vi "Begin.vi"(8 "error in":errorcluster) -> (0 "error out":errorcluster)   [LabVIEW 2019]
doc: "Called before other user functions, this VI is expected to open initial I/O refnums, load in file data, and do all program initialization. Notice that the <B>error out</B> terminal is simply used for data flow. Wiring it to other structures or subVIs ensures that this VI runs first."
uses:
  <vilib>/Rock Robotics/WPI/DriverStation/WPI_DriverStationRobotMode2.ctl
  <vilib>/Rock Robotics/WPI/Joystick/WPI_JoystickDeviceEnum.ctl
  <vilib>/Rock Robotics/SystemInterfaces/DIO/FPGA_DIOChannel.ctl
  <vilib>/Rock Robotics/WPI/Encoder/WPI_EncoderType.ctl
  <vilib>/Rock Robotics/WPI/ThirdParty/REV Robotics/SPARK MAX/Typedef/Spark MAX Motor Type.ctl
  <vilib>/Rock Robotics/WPI/ThirdParty/REV Robotics/SPARK MAX/Typedef/Spark MAX Idle Mode.ctl
  <vilib>/Rock Robotics/WPI/SafetyOutput/WPI_SafetyOutputConfigMenu.ctl
  <vilib>/Rock Robotics/WPI/ThirdParty/Phoenix-LabVIEW/Motor Controller/Controls/CTRE_Phoenix_MotorControl_ControlMode.ctl
  <vilib>/Rock Robotics/WPI/Solenoid/WPI_SolenoidChannel.ctl
  Robot Global Data.vi
  <vilib>/Rock Robotics/Network Tables/NT Write String Array.vi
  <vilib>/Rock Robotics/WPI/Counter/WPI_CounterDigitalInputToDigitalSource.vi
  <vilib>/Rock Robotics/WPI/RobotDrive/WPI_RobotDriveOpen4MotorWithExistingMotors.vi
  <vilib>/Rock Robotics/WPI/Solenoid/WPI_SolenoidOpenDouble.vi
  <vilib>/Rock Robotics/WPI/Switch/WPI_SwitchOpenLimit.vi
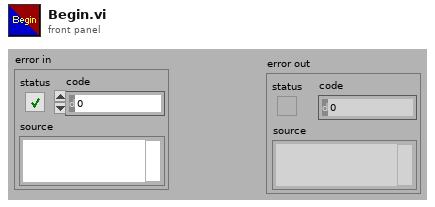
[diagram p1: front panel]
types:
  T1 = typedef "FPGA_DIOChannel.ctl" = enum8{"DIO 0", "DIO 1", "DIO 2", "DIO 3", "DIO 4", "DIO 5", "DIO 6", "DIO 7", "DIO 8", "DIO 9", "DIO MXP 0", "DIO MXP 1", "DIO MXP 2", "DIO MXP 3", "DIO MXP 4", "DIO MXP 5", "DIO MXP 6", "DIO MXP 7", "DIO MXP 8", "DIO MXP 9", "DIO MXP 10", "DIO MXP 11", "DIO MXP 12", "DIO MXP 13", "DIO MXP 14", "DIO MXP 15", "SPI Port CS1", "SPI Port CS2", "SPI Port CS3", "SPI Port MISO", "SPI Port MOSI", "Invalid"}
  T2 = typedef "CTRE_Phoenix_MotorControl_ControlMode.ctl" = u16
  T3 = typedef "WPI_SolenoidChannel.ctl" = enum8{"Solenoid 0", "Solenoid 1", "Solenoid 2", "Solenoid 3", "Solenoid 4", "Solenoid 5", "Solenoid 6", "Solenoid 7", "Invalid"}
  T4 = typedef "WPI_SafetyOutputConfigMenu.ctl" = enum16{"Enable", "Disable"}
  T5 = typedef "Spark MAX Idle Mode.ctl" = enum16{"Coast", "Brake"}
  T6 = typedef "Spark MAX Motor Type.ctl" = enum16{"Brushed", "Brushless"}
  T7 = typedef "WPI_EncoderType.ctl" = enum16{"1x", "2x", "4x"}
  T8 = typedef "WPI_JoystickDeviceEnum.ctl" = enum16{"USB 0", "USB 1", "USB 2", "USB 3", "USB 4", "USB 5"}
  T9 = typedef "WPI_DriverStationRobotMode2.ctl" = enum16{"Autonomous Disabled", "Autonomous Enabled", "Teleop Disabled", "Teleop Enabled", "Disconnected", "Finish", "Test Disabled", "Test Enabled", "Emergency Stopped"}
  T10 = typedef "WPI_SwitchDevRef.ctl" = cluster{"DevStatus":errorcluster, "DIO Channel":T1, "CntIndex":T11, "Normally Closed":bool}
  T11 = typedef "FPGA_CounterCtrSystemIndex.ctl" = enum8{"Ctr 0", "Ctr 1", "Ctr 2", "Ctr 3", "Ctr 4", "Ctr 5", "Ctr 6", "Ctr 7", "Invalid"}
  T12 = typedef "WPI_MotorControlDeviceRef.ctl" = cluster{"DeviceStatus":errorcluster, "Type":T13, "PWM":cluster{"PWM Channel":T14, "DeadBand":T15}, "CAN":cluster{"Device Number":u8, "SetOutput VI Ref":variant, "GetOutput VI Ref":variant, "Enable VI Ref":variant, "Disable VI Ref":variant, "Data":variant}, "Invert":bool, "DIO PWM":cluster{"PWM \"Enable\" Channel":T14, "DIOChannel":T1, "PWM Rate":dbl}}
  T13 = typedef "WPI_MotorControlType.ctl" = enum16{"PWM", "CAN", "DIO PWM"}
  T14 = typedef "FPGA_DIOPWMChannel.ctl" = enum8{"PWM 0", "PWM 1", "PWM 2", "PWM 3", "PWM 4", "PWM 5", "PWM 6", "PWM 7", "PWM 8", "PWM 9", "PWM MXP 0", "PWM MXP 1", "PWM MXP 2", "PWM MXP 3", "PWM MXP 4", "PWM MXP 5", "PWM MXP 6", "PWM MXP 7", "PWM MXP 8", "PWM MXP 9", "Invalid"}
  T15 = typedef "WPI_PWMDeadband.ctl" = cluster{"Name":string, "maxPositivePwm":i32, "minPositivePwm":i32, "centerPwm":i32, "maxNegativePwm":i32, "minNegativePwm":i32, "angularRange":u16}
  T16 = typedef "WPI_JoystickDevRef.ctl" = cluster{"Device":T8}
  T17 = typedef "WPI_RobotDriveDevRef.ctl" = cluster{"DevStatus":errorcluster, "Motors[]":T12[], "Square Inputs":bool, "Max Output":dbl}
  T18 = typedef "WPI_SolenoidDevRef.ctl" = cluster{"DevStatus":errorcluster, "Pneumatics Control Module":u8, "Forward Solenoid Channel":T3, "Reverse Solenoid Channel":T3}
  T19 = typedef "WPI_DigitalInputDevRef.ctl" = cluster{"DevStatus":errorcluster, "DIO Channel":T1}
  T20 = typedef "FPGA_CounterEncoderSourceConvertionLVSourceType.ctl" = cluster{"DevStatus":errorcluster, "AnalogTriggerMode?":bool, "DigitalMode":cluster{"DIO Channel":T21}, "AnalogTriggerMode":cluster{"AnalogTriggerIndex":T22, "OutputType":T23}}
  T21 = typedef "FPGA_DIODigitalSourceChannel.ctl" = enum8{"DIO 0", "DIO 1", "DIO 2", "DIO 3", "DIO 4", "DIO 5", "DIO 6", "DIO 7", "DIO 8", "DIO 9", "DIO MXP 0", "DIO MXP 1", "DIO MXP 2", "DIO MXP 3", "DIO MXP 4", "DIO MXP 5", "DIO MXP 6", "DIO MXP 7", "DIO MXP 8", "DIO MXP 9", "DIO MXP 10", "DIO MXP 11", "DIO MXP 12", "DIO MXP 13", "DIO MXP 14", "DIO MXP 15", "SPI Port CS1", "SPI Port CS2", "SPI Port CS3", "SPI Port MISO", "SPI Port MOSI", "Disabled"}
  T22 = typedef "FPGA_AnalogTriggerIndex.ctl" = enum8{"Trig 0", "Trig 1", "Trig 2", "Trig 3", "Trig 4", "Trig 5", "Trig 6", "Trig 7", "Invalid"}
  T23 = typedef "FPGA_AnalogTriggerOutType.ctl" = enum16{"InWindow", "TriggerState", "Rising", "Falling"}
  T24 = typedef "WPI_EncoderDevRef.ctl" = cluster{"DevStatus":errorcluster, "EncoderIndex":T25, "CounterIndex":T11, "DistancePerCount":dbl, "Decoding Type":T7}
  T25 = typedef "FPGA_EncoderIdx.ctl" = enum8{"Enc 0", "Enc 1", "Enc 2", "Enc 3", "Enc 4", "Enc 5", "Enc 6", "Enc 7", "Invalid"}
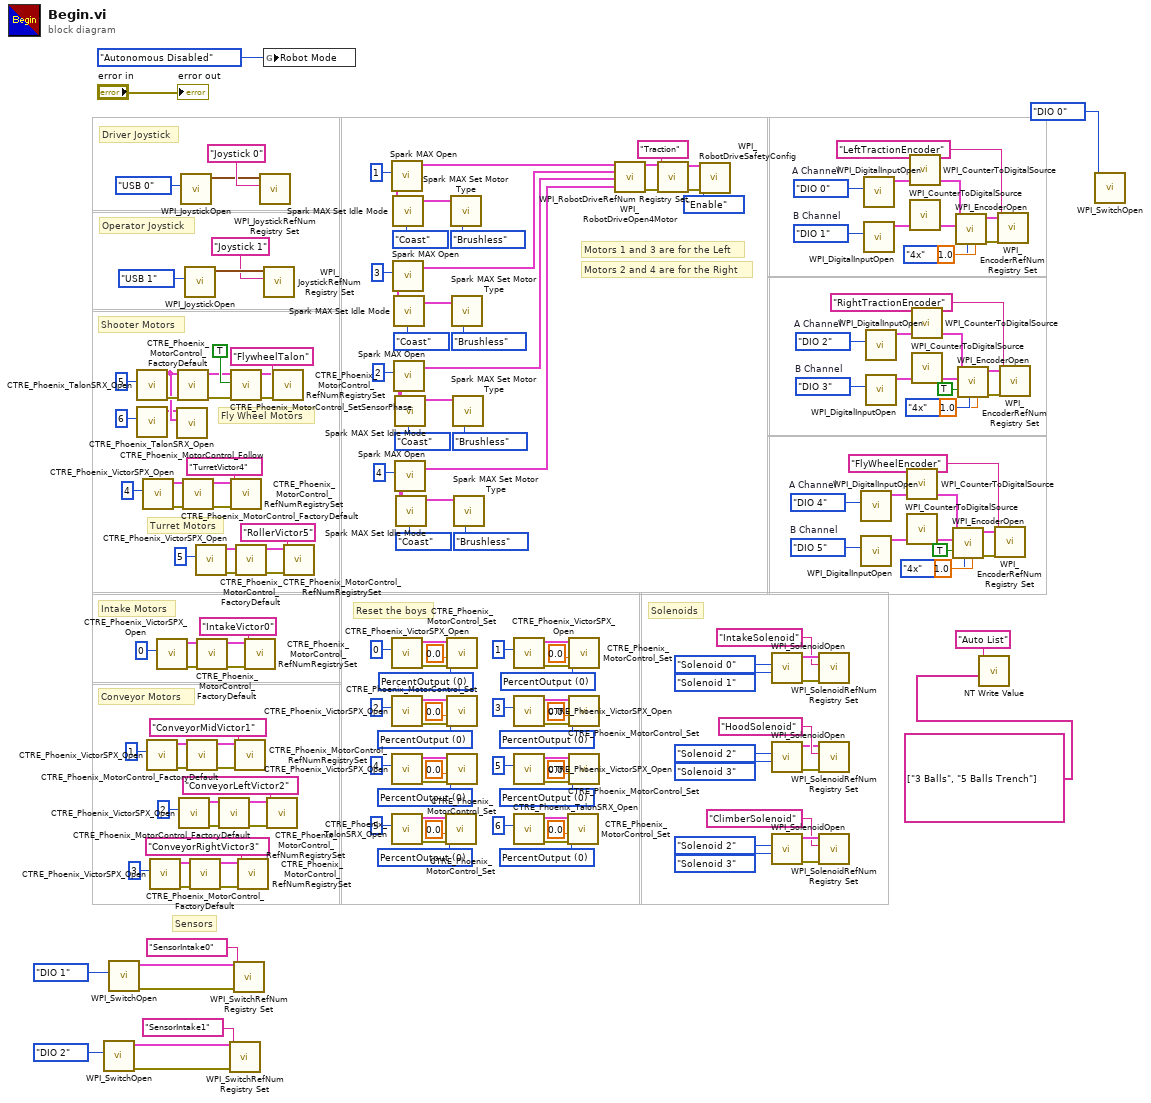
[diagram p0: block diagram]
diagram:
  w11 = T2 0 items=["PercentOutput"=0, "Position"=1, "Velocity"=2, "Current"=3, "Follower"=5, "MotionProfile"=6, "MotionMagic"=7, "MotionMagicArc"=8, "MotionProfileArc"=10, "Disabled"=15] ("Control Mode")
  w35 = T2 0 items=["PercentOutput"=0, "Position"=1, "Velocity"=2, "Current"=3, "Follower"=5, "MotionProfile"=6, "MotionMagic"=7, "MotionMagicArc"=8, "MotionProfileArc"=10, "Disabled"=15] ("Control Mode")
  w41 = T2 0 items=["PercentOutput"=0, "Position"=1, "Velocity"=2, "Current"=3, "Follower"=5, "MotionProfile"=6, "MotionMagic"=7, "MotionMagicArc"=8, "MotionProfileArc"=10, "Disabled"=15] ("Control Mode")
  w40 = T2 0 items=["PercentOutput"=0, "Position"=1, "Velocity"=2, "Current"=3, "Follower"=5, "MotionProfile"=6, "MotionMagic"=7, "MotionMagicArc"=8, "MotionProfileArc"=10, "Disabled"=15] ("Control Mode")
  w50 = T2 0 items=["PercentOutput"=0, "Position"=1, "Velocity"=2, "Current"=3, "Follower"=5, "MotionProfile"=6, "MotionMagic"=7, "MotionMagicArc"=8, "MotionProfileArc"=10, "Disabled"=15] ("Control Mode")
  w51 = T2 0 items=["PercentOutput"=0, "Position"=1, "Velocity"=2, "Current"=3, "Follower"=5, "MotionProfile"=6, "MotionMagic"=7, "MotionMagicArc"=8, "MotionProfileArc"=10, "Disabled"=15] ("Control Mode")
  w60 = T2 0 items=["PercentOutput"=0, "Position"=1, "Velocity"=2, "Current"=3, "Follower"=5, "MotionProfile"=6, "MotionMagic"=7, "MotionMagicArc"=8, "MotionProfileArc"=10, "Disabled"=15] ("Control Mode")
  w61 = T2 0 items=["PercentOutput"=0, "Position"=1, "Velocity"=2, "Current"=3, "Follower"=5, "MotionProfile"=6, "MotionMagic"=7, "MotionMagicArc"=8, "MotionProfileArc"=10, "Disabled"=15] ("Control Mode")
  w145 = FPGA_DIOChannel."DIO 5"  # B Channel
  w144 = FPGA_DIOChannel."DIO 4"  # A Channel
  w148 = FPGA_DIOChannel."DIO 3"  # B Channel
  w149 = FPGA_DIOChannel."DIO 2"  # A Channel
  w169 = FPGA_DIOChannel."DIO 1"  # B Channel
  w168 = FPGA_DIOChannel."DIO 0"  # A Channel
  # "Sensors"
  # "Solenoids"
  # "Reset the boys"
  # "Conveyor Motors"
  # "Intake Motors"
  # "Turret Motors"
  # "Fly Wheel Motors"
  # "Shooter Motors"
  # "Motors 2 and 4 are for the Right"
  # "Motors 1 and 3 are for the Left"
  # "Operator Joystick"
  # "Driver Joystick"
  n1 = call-poly <vilib>:"WPI_SwitchOpen.vi"("DIO Channel"=FPGA_DIOChannel."DIO 2") -> ("error out"=w5:errorcluster, "SwitchDevRef"=w4:T10)  [unwired: 9 in]
  n2 = call-poly <vilib>:"WPI_SwitchOpen.vi"("DIO Channel"=FPGA_DIOChannel."DIO 1") -> ("error out"=w7:errorcluster, "SwitchDevRef"=w8:T10)  [unwired: 9 in]
  n3 = call <vilib>:"CTRE_Phoenix_TalonSRX_Open.vi"("Device Number"=u8 5) -> ("error out"=w105:errorcluster, "CAN Talon SRX Ref"=w104:T12)  [unwired: 9 in]
  n4 = call <vilib>:"CTRE_Phoenix_TalonSRX_Open.vi"("Device Number"=u8 6) -> ("CAN Talon SRX Ref"=w67:T12)  [unwired: 9 in, 1 out]
  n5 = call <vilib>:"CTRE_Phoenix_VictorSPX_Open.vi"("Device Number"=u8 4) -> ("error out"=w79:errorcluster, "CAN Talon SRX Ref"=w78:T12)  [unwired: 9 in]
  n6 = call <vilib>:"CTRE_Phoenix_VictorSPX_Open.vi"("Device Number"=u8 1) -> ("error out"=w92:errorcluster, "CAN Talon SRX Ref"=w93:T12)  [unwired: 9 in]
  n7 = call <vilib>:"CTRE_Phoenix_VictorSPX_Open.vi"("Device Number"=u8 3) -> ("error out"=w80:errorcluster, "CAN Talon SRX Ref"=w81:T12)  [unwired: 9 in]
  n8 = call <vilib>:"CTRE_Phoenix_VictorSPX_Open.vi"("Device Number"=u8 0) -> ("error out"=w103:errorcluster, "CAN Talon SRX Ref"=w102:T12)  [unwired: 9 in]
  n9 = call <vilib>:"CTRE_Phoenix_MotorControl_Follow.vi"("Master Controller to Follow"=w104, "PhoenixMotorControlDevRef"=w67) -> ()  [unwired: 8 in, 2 out]
  n10 = call <vilib>:"CTRE_Phoenix_MotorControl_FactoryDefault.vi"("error in"=w105, "PhoenixMotorControlDevRef"=w104) -> ("error out"=w108:errorcluster, "PhoenixMotorControlDevRef"=w109:T12)  [unwired: 8 in]
  n11 = call <vilib>:"CTRE_Phoenix_VictorSPX_Open.vi"("Device Number"=u8 2) -> ("error out"=w91:errorcluster, "CAN Talon SRX Ref"=w90:T12)  [unwired: 9 in]
  n12 = call <vilib>:"WPI_JoystickOpen.vi"("JoystickDevice"=WPI_JoystickDeviceEnum."USB 0") -> ("JoystickDevRef"=w176:T16)  [unwired: 10 in]
  n13 = call <vilib>:"CTRE_Phoenix_MotorControl_FactoryDefault.vi"("error in"=w79, "PhoenixMotorControlDevRef"=w78) -> ("error out"=w77:errorcluster, "PhoenixMotorControlDevRef"=w75:T12)  [unwired: 8 in]
  n14 = call <vilib>:"WPI_JoystickOpen.vi"("JoystickDevice"=WPI_JoystickDeviceEnum."USB 1") -> ("JoystickDevRef"=w171:T16)  [unwired: 10 in]
  n15 = call <vilib>:"CTRE_Phoenix_MotorControl_FactoryDefault.vi"("error in"=w92, "PhoenixMotorControlDevRef"=w93) -> ("error out"=w94:errorcluster, "PhoenixMotorControlDevRef"=w95:T12)  [unwired: 8 in]
  n16 = call <vilib>:"CTRE_Phoenix_MotorControl_FactoryDefault.vi"("error in"=w80, "PhoenixMotorControlDevRef"=w81) -> ("error out"=w82:errorcluster, "PhoenixMotorControlDevRef"=w83:T12)  [unwired: 8 in]
  n17 = call <vilib>:"CTRE_Phoenix_VictorSPX_Open.vi"("Device Number"=u8 5) -> ("error out"=w68:errorcluster, "CAN Talon SRX Ref"=w69:T12)  [unwired: 9 in]
  n18 = call <vilib>:"CTRE_Phoenix_MotorControl_FactoryDefault.vi"("error in"=w103, "PhoenixMotorControlDevRef"=w102) -> ("error out"=w101:errorcluster, "PhoenixMotorControlDevRef"=w100:T12)  [unwired: 8 in]
  n19 = call <vilib>:"CTRE_Phoenix_MotorControl_FactoryDefault.vi"("error in"=w91, "PhoenixMotorControlDevRef"=w90) -> ("error out"=w89:errorcluster, "PhoenixMotorControlDevRef"=w88:T12)  [unwired: 8 in]
  n20 = call <vilib>:"WPI_SwitchRefNum Registry Set.vi"("error in (no error)"=w5, "refnum name"="SensorIntake1", "SwitchDevRef"=w4) -> ()  [unwired: 7 in, 2 out]
  n21 = call <vilib>:"CTRE_Phoenix_MotorControl_SetSensorPhase.vi"("error in (no error)"=w108, "PhaseSensor"=TRUE, "PhoenixMotorControlDevRef"=w109) -> ("error out"=w106:errorcluster, "PhoenixMotorControlDevRef"=w107:T12)  [unwired: 7 in]
  n22 = call <vilib>:"CTRE_Phoenix_MotorControl_RefNumRegistrySet.vi"("error in (no error)"=w77, "refnum name"="TurretVictor4", "PhoenixMotorControlDevRef"=w75) -> ()  [unwired: 7 in, 2 out]
  n23 = call <vilib>:"WPI_SwitchRefNum Registry Set.vi"("error in (no error)"=w7, "refnum name"="SensorIntake0", "SwitchDevRef"=w8) -> ()  [unwired: 7 in, 2 out]
  n24 = call <vilib>:"CTRE_Phoenix_MotorControl_RefNumRegistrySet.vi"("error in (no error)"=w94, "refnum name"="ConveyorMidVictor1", "PhoenixMotorControlDevRef"=w95) -> ()  [unwired: 7 in, 2 out]
  n25 = call <vilib>:"CTRE_Phoenix_MotorControl_FactoryDefault.vi"("error in"=w68, "PhoenixMotorControlDevRef"=w69) -> ("error out"=w70:errorcluster, "PhoenixMotorControlDevRef"=w72:T12)  [unwired: 8 in]
  n26 = call <vilib>:"CTRE_Phoenix_MotorControl_RefNumRegistrySet.vi"("error in (no error)"=w82, "refnum name"="ConveyorRightVictor3", "PhoenixMotorControlDevRef"=w83) -> ()  [unwired: 7 in, 2 out]
  n27 = call <vilib>:"CTRE_Phoenix_MotorControl_RefNumRegistrySet.vi"("error in (no error)"=w101, "refnum name"="IntakeVictor0", "PhoenixMotorControlDevRef"=w100) -> ()  [unwired: 7 in, 2 out]
  n28 = call <vilib>:"WPI_JoystickRefNum Registry Set.vi"("refnum name"="Joystick 0", "JoystickDevRef"=w176) -> ()  [unwired: 8 in, 2 out]
  n29 = global write "Robot Global Data.vi" "Robot Mode"(WPI_DriverStationRobotMode2."Autonomous Disabled" ("Robot Mode")) -> ()
  n30 = call <vilib>:"WPI_JoystickRefNum Registry Set.vi"("refnum name"="Joystick 1", "JoystickDevRef"=w171) -> ()  [unwired: 8 in, 2 out]
  n31 = call <vilib>:"CTRE_Phoenix_MotorControl_RefNumRegistrySet.vi"("error in (no error)"=w89, "refnum name"="ConveyorLeftVictor2", "PhoenixMotorControlDevRef"=w88) -> ()  [unwired: 7 in, 2 out]
  n32 = call <vilib>:"CTRE_Phoenix_MotorControl_RefNumRegistrySet.vi"("error in (no error)"=w106, "refnum name"="FlywheelTalon", "PhoenixMotorControlDevRef"=w107) -> ()  [unwired: 7 in, 2 out]
  n33 = call <vilib>:"CTRE_Phoenix_MotorControl_RefNumRegistrySet.vi"("error in (no error)"=w70, "refnum name"="RollerVictor5", "PhoenixMotorControlDevRef"=w72) -> ()  [unwired: 7 in, 2 out]
  n34 = call <vilib>:"Spark MAX Open.vi"("Device Number"=u8 1) -> ("MotorControlDeviceRef"=w131:T12)  [unwired: 9 in, 1 out]
  n35 = call <vilib>:"CTRE_Phoenix_VictorSPX_Open.vi"("Device Number"=u8 0) -> ("error out"=w55:errorcluster, "CAN Talon SRX Ref"=w54:T12)  [unwired: 9 in]
  n36 = call <vilib>:"CTRE_Phoenix_VictorSPX_Open.vi"("Device Number"=u8 2) -> ("error out"=w46:errorcluster, "CAN Talon SRX Ref"=w47:T12)  [unwired: 9 in]
  n37 = call <vilib>:"CTRE_Phoenix_VictorSPX_Open.vi"("Device Number"=u8 4) -> ("error out"=w31:errorcluster, "CAN Talon SRX Ref"=w32:T12)  [unwired: 9 in]
  n38 = call <vilib>:"CTRE_Phoenix_TalonSRX_Open.vi"("Device Number"=u8 5) -> ("error out"=w65:errorcluster, "CAN Talon SRX Ref"=w64:T12)  [unwired: 9 in]
  n39 = call <vilib>:"Spark MAX Set Idle Mode.vi"("Idle Mode"=Spark_MAX_Idle_Mode."Coast", "MotorControlDeviceRef in"=w131) -> ()  [unwired: 8 in, 2 out]
  n40 = call <vilib>:"Spark MAX Open.vi"("Device Number"=u8 3) -> ("MotorControlDeviceRef"=w127:T12)  [unwired: 9 in, 1 out]
  n41 = call <vilib>:"Spark MAX Set Idle Mode.vi"("Idle Mode"=Spark_MAX_Idle_Mode."Coast", "MotorControlDeviceRef in"=w127) -> ()  [unwired: 8 in, 2 out]
  n42 = call <vilib>:"Spark MAX Open.vi"("Device Number"=u8 2) -> ("MotorControlDeviceRef"=w123:T12)  [unwired: 9 in, 1 out]
  n43 = call <vilib>:"Spark MAX Set Idle Mode.vi"("Idle Mode"=Spark_MAX_Idle_Mode."Coast", "MotorControlDeviceRef in"=w123) -> ()  [unwired: 8 in, 2 out]
  n44 = call <vilib>:"Spark MAX Open.vi"("Device Number"=u8 4) -> ("MotorControlDeviceRef"=w119:T12)  [unwired: 9 in, 1 out]
  n45 = call <vilib>:"Spark MAX Set Idle Mode.vi"("Idle Mode"=Spark_MAX_Idle_Mode."Coast", "MotorControlDeviceRef in"=w119) -> ()  [unwired: 8 in, 2 out]
  n46 = call <vilib>:"CTRE_Phoenix_MotorControl_Set.vi"("error in (no error)"=w65, "Output"=0.0, "Control Mode"=w61, "PhoenixMotorControlDevRef"=w64) -> ()  [unwired: 6 in, 2 out]
  n47 = call <vilib>:"CTRE_Phoenix_MotorControl_Set.vi"("error in (no error)"=w55, "Output"=0.0, "Control Mode"=w51, "PhoenixMotorControlDevRef"=w54) -> ()  [unwired: 6 in, 2 out]
  n48 = call <vilib>:"CTRE_Phoenix_MotorControl_Set.vi"("error in (no error)"=w46, "Output"=0.0, "Control Mode"=w50, "PhoenixMotorControlDevRef"=w47) -> ()  [unwired: 6 in, 2 out]
  n49 = call <vilib>:"CTRE_Phoenix_MotorControl_Set.vi"("error in (no error)"=w31, "Output"=0.0, "Control Mode"=w35, "PhoenixMotorControlDevRef"=w32) -> ()  [unwired: 6 in, 2 out]
  n50 = call <vilib>:"Spark MAX Set Motor Type.vi"("Motor Type"=Spark_MAX_Motor_Type."Brushless", "MotorControlDevRef"=w131) -> ()  [unwired: 8 in, 2 out]
  n51 = call <vilib>:"Spark MAX Set Motor Type.vi"("Motor Type"=Spark_MAX_Motor_Type."Brushless", "MotorControlDevRef"=w127) -> ()  [unwired: 8 in, 2 out]
  n52 = call <vilib>:"Spark MAX Set Motor Type.vi"("Motor Type"=Spark_MAX_Motor_Type."Brushless", "MotorControlDevRef"=w123) -> ()  [unwired: 8 in, 2 out]
  n53 = call <vilib>:"Spark MAX Set Motor Type.vi"("Motor Type"=Spark_MAX_Motor_Type."Brushless", "MotorControlDevRef"=w119) -> ()  [unwired: 8 in, 2 out]
  n54 = call <vilib>:"CTRE_Phoenix_VictorSPX_Open.vi"("Device Number"=u8 1) -> ("error out"=w36:errorcluster, "CAN Talon SRX Ref"=w37:T12)  [unwired: 9 in]
  n55 = call <vilib>:"CTRE_Phoenix_VictorSPX_Open.vi"("Device Number"=u8 3) -> ("error out"=w45:errorcluster, "CAN Talon SRX Ref"=w44:T12)  [unwired: 9 in]
  n56 = call <vilib>:"CTRE_Phoenix_VictorSPX_Open.vi"("Device Number"=u8 5) -> ("error out"=w14:errorcluster, "CAN Talon SRX Ref"=w9:T12)  [unwired: 9 in]
  n57 = call <vilib>:"CTRE_Phoenix_TalonSRX_Open.vi"("Device Number"=u8 6) -> ("error out"=w56:errorcluster, "CAN Talon SRX Ref"=w57:T12)  [unwired: 9 in]
  n58 = call <vilib>:"CTRE_Phoenix_MotorControl_Set.vi"("error in (no error)"=w56, "Output"=0.0, "Control Mode"=w60, "PhoenixMotorControlDevRef"=w57) -> ()  [unwired: 6 in, 2 out]
  n59 = call <vilib>:"CTRE_Phoenix_MotorControl_Set.vi"("error in (no error)"=w36, "Output"=0.0, "Control Mode"=w40, "PhoenixMotorControlDevRef"=w37) -> ()  [unwired: 6 in, 2 out]
  n60 = call <vilib>:"CTRE_Phoenix_MotorControl_Set.vi"("error in (no error)"=w45, "Output"=0.0, "Control Mode"=w41, "PhoenixMotorControlDevRef"=w44) -> ()  [unwired: 6 in, 2 out]
  n61 = call <vilib>:"CTRE_Phoenix_MotorControl_Set.vi"("error in (no error)"=w14, "Output"=0.0, "Control Mode"=w11, "PhoenixMotorControlDevRef"=w9) -> ()  [unwired: 6 in, 2 out]
  n62 = call-poly <vilib>:"WPI_RobotDriveOpen4Motor.vi"("Rear Left Motor Dev Ref"=w131, "Rear Right Motor Dev Ref"=w127, "Front Left Motor Dev Ref"=w123, "Front Right Motor Dev Ref"=w119) -> ("RobotDriveDevRef"=w117:T17, "error out"=w118:errorcluster)  [unwired: 10 in]
  n63 = call <vilib>:"WPI_RobotDriveRefNum Registry Set.vi"("error in (no error)"=w118, "refnum name"="Traction", "RobotDriveDevRef"=w117) -> ("error out"=w115:errorcluster, "RobotDriveDevRef"=w114:T17)  [unwired: 7 in]
  n64 = call <vilib>:"WPI_RobotDriveSafetyConfig.vi"("error in (no error)"=w115, "mode"=WPI_SafetyOutputConfigMenu."Enable", "RobotDriveDevRef"=w114) -> ()  [unwired: 7 in, 2 out]
  n65 = call-poly <vilib>:"WPI_SolenoidOpen.vi"("Reverse Solenoid Channel"=WPI_SolenoidChannel."Solenoid 1", "Forward Solenoid Channel"=WPI_SolenoidChannel."Solenoid 0") -> ("error out"=w30:errorcluster, "SolenoidDevRef"=w29:T18)  [unwired: 8 in]
  n66 = call-poly <vilib>:"WPI_SolenoidOpen.vi"("Reverse Solenoid Channel"=WPI_SolenoidChannel."Solenoid 3", "Forward Solenoid Channel"=WPI_SolenoidChannel."Solenoid 2") -> ("error out"=w21:errorcluster, "SolenoidDevRef"=w22:T18)  [unwired: 8 in]
  n67 = call-poly <vilib>:"WPI_SolenoidOpen.vi"("Reverse Solenoid Channel"=WPI_SolenoidChannel."Solenoid 3", "Forward Solenoid Channel"=WPI_SolenoidChannel."Solenoid 2") -> ("error out"=w20:errorcluster, "SolenoidDevRef"=w19:T18)  [unwired: 8 in]
  n68 = call <vilib>:"WPI_SolenoidRefNum Registry Set.vi"("error in (no error)"=w30, "refnum name"="IntakeSolenoid", "SolenoidDevRef"=w29) -> ()  [unwired: 7 in, 2 out]
  n69 = call <vilib>:"WPI_SolenoidRefNum Registry Set.vi"("error in (no error)"=w21, "refnum name"="HoodSolenoid", "SolenoidDevRef"=w22) -> ()  [unwired: 7 in, 2 out]
  n70 = call <vilib>:"WPI_SolenoidRefNum Registry Set.vi"("error in (no error)"=w20, "refnum name"="ClimberSolenoid", "SolenoidDevRef"=w19) -> ()  [unwired: 7 in, 2 out]
  n71 = call <vilib>:"WPI_DigitalInputOpen.vi"("DIO Channel"=w144) -> ("DigitalInputDevRef"=w141:T19)  [unwired: 1 in, 9 out]
  n72 = call <vilib>:"WPI_DigitalInputOpen.vi"("DIO Channel"=w145) -> ("DigitalInputDevRef"=w142:T19)  [unwired: 1 in, 9 out]
  n73 = call <vilib>:"WPI_DigitalInputOpen.vi"("DIO Channel"=w168) -> ("DigitalInputDevRef"=w165:T19)  [unwired: 1 in, 9 out]
  n74 = call <vilib>:"WPI_DigitalInputOpen.vi"("DIO Channel"=w169) -> ("DigitalInputDevRef"=w166:T19)  [unwired: 1 in, 9 out]
  n75 = call <vilib>:"WPI_DigitalInputOpen.vi"("DIO Channel"=w149) -> ("DigitalInputDevRef"=w152:T19)  [unwired: 1 in, 9 out]
  n76 = call <vilib>:"WPI_DigitalInputOpen.vi"("DIO Channel"=w148) -> ("DigitalInputDevRef"=w151:T19)  [unwired: 1 in, 9 out]
  n77 = call-poly <vilib>:"WPI_CounterToDigitalSource.vi"("DigitalInputDevRef"=w141) -> ("Digital Source"=w140:T20)  [unwired: 6 out]
  n78 = call-poly <vilib>:"WPI_CounterToDigitalSource.vi"("DigitalInputDevRef"=w142) -> ("Digital Source"=w143:T20)  [unwired: 6 out]
  n79 = call-poly <vilib>:"WPI_CounterToDigitalSource.vi"("DigitalInputDevRef"=w165) -> ("Digital Source"=w164:T20)  [unwired: 6 out]
  n80 = call-poly <vilib>:"WPI_CounterToDigitalSource.vi"("DigitalInputDevRef"=w166) -> ("Digital Source"=w167:T20)  [unwired: 6 out]
  n81 = call-poly <vilib>:"WPI_CounterToDigitalSource.vi"("DigitalInputDevRef"=w152) -> ("Digital Source"=w153:T20)  [unwired: 6 out]
  n82 = call-poly <vilib>:"WPI_CounterToDigitalSource.vi"("DigitalInputDevRef"=w151) -> ("Digital Source"=w150:T20)  [unwired: 6 out]
  n83 = call <vilib>:"WPI_EncoderOpen.vi"("DistancePerCount"=1.0, "Decoding Type"=WPI_EncoderType."4x", "Invert Direction (False)"=TRUE, "BSource"=w143, "ASource"=w140) -> ("error out"=w137:errorcluster, "EncoderDevRef"=w136:T24)  [unwired: 3 in, 2 out]
  n84 = call <vilib>:"WPI_EncoderOpen.vi"("DistancePerCount"=1.0, "Decoding Type"=WPI_EncoderType."4x", "BSource"=w167, "ASource"=w164) -> ("error out"=w161:errorcluster, "EncoderDevRef"=w160:T24)  [unwired: 4 in, 2 out]
  n85 = call <vilib>:"WPI_EncoderOpen.vi"("DistancePerCount"=1.0, "Decoding Type"=WPI_EncoderType."4x", "Invert Direction (False)"=TRUE, "BSource"=w150, "ASource"=w153) -> ("error out"=w156:errorcluster, "EncoderDevRef"=w157:T24)  [unwired: 3 in, 2 out]
  n86 = call-poly <vilib>:"NT Write Value.vi"("String Array"=string[] ["3 Balls", "5 Balls Trench"], "Name"="Auto List") -> ()  [unwired: 9 in, 1 out]
  n87 = call <vilib>:"WPI_EncoderRefNum Registry Set.vi"("error in (no error)"=w137, "refnum name"="FlyWheelEncoder", "EncoderDevRef"=w136) -> ()  [unwired: 7 in, 2 out]
  n88 = call <vilib>:"WPI_EncoderRefNum Registry Set.vi"("error in (no error)"=w161, "refnum name"="LeftTractionEncoder", "EncoderDevRef"=w160) -> ()  [unwired: 7 in, 2 out]
  n89 = call <vilib>:"WPI_EncoderRefNum Registry Set.vi"("error in (no error)"=w156, "refnum name"="RightTractionEncoder", "EncoderDevRef"=w157) -> ()  [unwired: 7 in, 2 out]
  n90 = call-poly <vilib>:"WPI_SwitchOpen.vi"("DIO Channel"=FPGA_DIOChannel."DIO 0") -> ()  [unwired: 9 in, 2 out]
  "error out" <- "error in"
